vi "Get Command Format String.vi"(1 "Command":string="connect", 7 "Parameters":T1[](array[typedef])=[{"Name"="Instance", "Type"=enum."decimal"}, {"Name"="host", "Type"=enum."string"}, {"Name"="port", "Type"=enum."decimal"}]) -> (8 "Command Format String":string="connect Instance=%s; host=%d; port=%s; ")   [LabVIEW 2012]
uses:
  Controls/Parameter.ctl
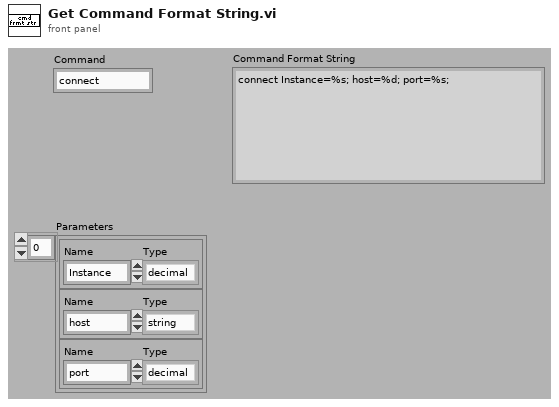
[diagram p1: front panel]
types:
  T1 = typedef "Parameter.ctl" = cluster{"Name":string, "Type":enum16{"decimal", "string", "float", "hex"}}
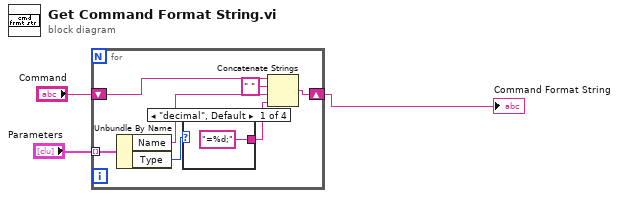
[diagram p0: block diagram]
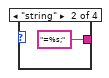
[diagram p2: hidden frame]
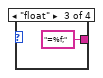
[diagram p3: hidden frame]
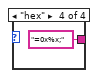
[diagram p4: hidden frame]
diagram:
  n1 = for {
    tunnel: "Parameters" -> [w10] mode=indexing
    shift-right: [w6] -> w1
    shift-left: "Command" -> [w5]
    n2 = Unbundle By Name(w10) -> ("Name"=w8:string, "Type"=w9:enum16{"decimal", "string", "float", "hex"})
    n3 = case shown="\"decimal\", Default" w9 {
      tunnel: ["=%d;" ("format string") "=%s;" ("format string") "=%f;" ("format string") "=0x%x;" ("format string")] -> w7
      frame "decimal", Default {
      }
      frame "string" {
      }
      frame "float" {
      }
      frame "hex" {
      }
    }
    n4 = Concatenate Strings(w5, " " ("string"), w8, w7) -> (w6:string)
  }
  "Command Format String" <- w1
